vi "Build Socket CAN.vi"(4 "Interface Mode":T1=enum."CAN FD BRS", 6 "extended?":bool=TRUE, 7 "TAI Time (ns)":i64, 8 "error in (no error)":errorcluster, 9 "Payload":u8[](array[numeric])=[10, 11, 10, 13, 11, 10, 11, 14] format="%.0x", 10 "identifier":u32=9 format="%.0x", 11 "pcap Parse and Build in":refnum<class "pcap_Parse_Build_CIF.lvclass">) -> (0 "error out":errorcluster, 2 "CAN Packet":u8[](array[numeric]), 3 "pcap Parse and Build out":refnum<class "pcap_Parse_Build_CIF.lvclass">)   [LabVIEW 2021, in "pcap_Parse_Build_CIF.lvclass"]
uses:
  pcap_Parse_Build_CIF.lvclass
  Typedef/Socket CAN Header.ctl
  pcap_Parse_Build_CIF.lvclass/pcap_Parse_Build_CIF.ctl
  <vilib>/CIF Foundation/CIF Utilities/Time/System Time/LabVIEW Time to TAI Time.vi
  Build/SubVIs/Flatten SocketCAN Header.vi/e4177ba7-55c0-4140-bea2-15e5e44a53d0.vi
  Build/SubVIs/Flatten Packet Header.vi
  Build/SubVIs/Flatten SocketCAN Header.vi/e4177ba7-55c0-4140-bea2-15e5e44a53d0.vi/c28b0ead-42ad-4072-80a2-aca7f2bd7ce3.vi
  Build/SubVIs/Flatten Packet Header.vi/e4177ba7-55c0-4140-bea2-15e5e44a53d0.vi
  Build/SubVIs/Flatten Packet Header.vi/e4177ba7-55c0-4140-bea2-15e5e44a53d0.vi/c28b0ead-42ad-4072-80a2-aca7f2bd7ce3.vi
  Typedef/CAN Interface Mode.ctl
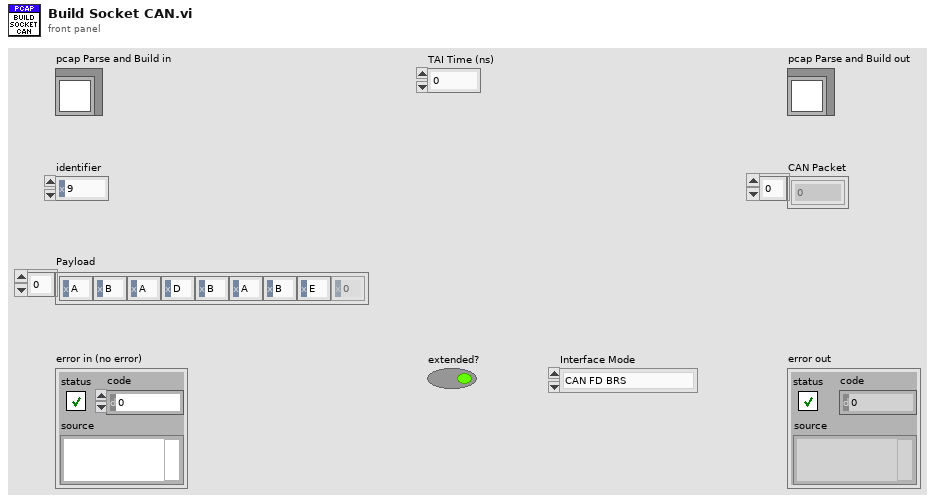
[diagram p1: front panel]
types:
  T1 = typedef "pcap_Parse_Build_CIF.lvclass/CAN Interface Mode.ctl" = enum16{"CAN 2.0", "CAN FD", "CAN FD BRS", "Remote"}
  T2 = typedef "pcap_Parse_Build_CIF.lvclass/Socket CAN Header.ctl" = cluster{"CANID and Flags":u32, "Payload Length":u8, "FD Flags":u8, "RSVD":u8, "Len8 DLC":u8}
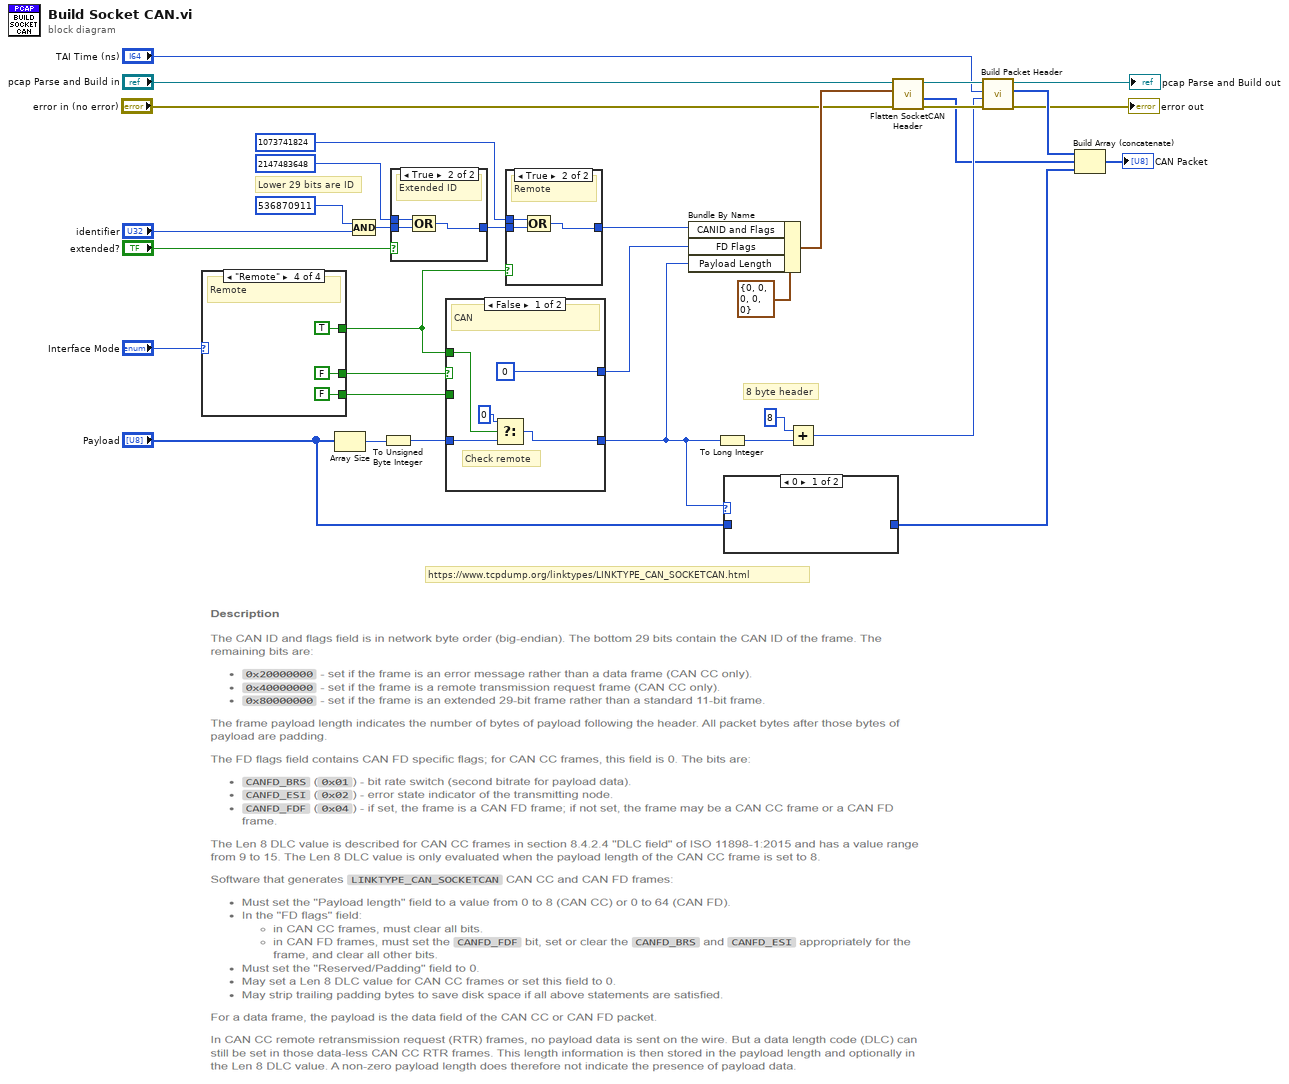
[diagram p0: block diagram]
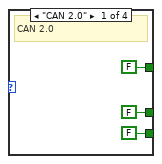
[diagram p3: hidden frame]
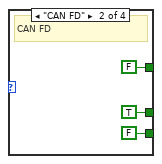
[diagram p4: hidden frame]
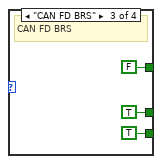
[diagram p5: hidden frame]
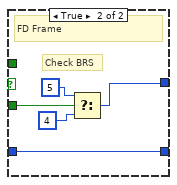
[diagram p8: hidden frame]
diagram:
  # "8 byte header"
  # "Lower 29 bits are ID"
  # "https://www.tcpdump.org/linktypes/LINKTYPE_CAN_SOCKETCAN.html"
  n1 = case shown="\"Remote\"" "Interface Mode" {
    tunnel: [FALSE FALSE FALSE TRUE] -> w21
    tunnel: [FALSE TRUE TRUE FALSE] -> w18
    tunnel: [FALSE FALSE TRUE FALSE] -> w19
    frame "CAN 2.0" {
      # "CAN 2.0"
    }
    frame "CAN FD" {
      # "CAN FD"
    }
    frame "CAN FD BRS" {
      # "CAN FD BRS"
    }
    frame "Remote" {
      # "Remote"
    }
  }
  n2 = Array Size(array="Payload") -> (size(s)=w22:i32)
  n3 = Compound Arithmetic op=AND(u32 536870911 ("number"), "identifier") -> (w28:u32)
  n4 = To Unsigned Byte Integer(number=w22) -> (unsigned 8bit integer=w20:u8)
  n5 = case shown="True" "extended?" {
    tunnel: w28 -> [w46 w49]
    tunnel: u32 2147483648 -> [_ w48]
    tunnel: [w46 w47] -> w26
    frame False {
    }
    frame True {
      # "Extended ID"
      n6 = Compound Arithmetic op=OR(w48, w49) -> (w47:u32)
    }
  }
  n7 = case shown="False" w18 {
    tunnel: w19 -> [_ w58]
    tunnel: [u8 0 w55] -> w23
    tunnel: w20 -> [w53 w59]
    tunnel: [w50 w59] -> w9
    tunnel: w21 -> [w52 _]
    frame False {
      # "Check remote"
      # "CAN"
      n8 = Select(t=u8 0, s=w52, f=w53) -> (s? t:f=w50:u8)
    }
    frame True {
      # "Check BRS"
      # "FD Frame"
      n9 = Select(t=u8 5, s=w58, f=u8 4) -> (s? t:f=w55:u8)
    }
  }
  n10 = case shown="True" w21 {
    tunnel: w26 -> [w60 w63]
    tunnel: [w60 w62] -> w24
    tunnel: u32 1073741824 -> [_ w61]
    frame False {
    }
    frame True {
      # "Remote"
      n11 = Compound Arithmetic op=OR(w61, w63) -> (w62:u32)
    }
  }
  n12 = Bundle By Name(cluster=T2 {"CANID and Flags"=0, "Payload Length"=0, "FD Flags"=0, "RSVD"=0, "Len8 DLC"=0} ("CAN Header out 2"), "CANID and Flags"=w24, "FD Flags"=w23, "Payload Length"=w9) -> (w11:T2)
  n13 = To Long Integer(number=w9) -> (32bit integer=w16:i32)
  n14 = case shown="0" w9 {
    tunnel: "Payload" -> [_ w64]
    tunnel: [_ w64] -> w7
    frame 0 {
    }
    frame 1, Default {
    }
  }
  n15 = Add(x=8, y=w16) -> (x+y=w10:i32)
  n16 = call "Flatten SocketCAN Header.vi"("error in (no error)"="error in (no error)", "CAN Header in"=w11, "pcap Parse and Build in"="pcap Parse and Build in") -> ("error out"=w30:errorcluster, "Flattened Data out"=w5:u8[], "pcap Parse and Build out"=w31:refnum<class "pcap_Parse_Build_CIF.lvclass">)  [unwired: 5 in, 1 out]
  n17 = call "Build Packet Header.vi"("error in (no error)"=w30, "Length"=w10, "TAI Time (ns)"="TAI Time (ns)", "pcap Parse and Build in"=w31) -> ("error out"=→"error out":errorcluster, "Flattened Data out"=w6:u8[], "pcap Parse and Build out"=→"pcap Parse and Build out":refnum<class "pcap_Parse_Build_CIF.lvclass">)  [unwired: 5 in]
  n18 = Build Array (concatenate)(w6, w5, w7) -> (→"CAN Packet":u8[])
